vi "Lambda Genesys Initialization VI.vi"(8 "error in (no error)":errorcluster, 10 "Custom XML":string, 11 "Device Item Ref in":T1 format="%.0x") -> (0 "error out":errorcluster, 3 "Device Item Ref out":T1 format="%.0x")   [LabVIEW 2011, in "Lambda Genesys2 Custom Device.lvlib"]
doc: "The Initialization VI is used to populate the tree with the most important elements. It is mandatory to add at least the main page!\nBy calling the Add Items VI make sure that sections are added before the channels. Also make sure that for nested sections each individual section is created (from top to bottwom)."
uses:
  Lambda Genesys2 Custom Device.lvlib
  <vilib>/NI Veristand/Custom Device API/Custom Device Item Ref.ctl
  <vilib>/NI Veristand/Custom Device API/Custom Device Channel.ctl
  <vilib>/NI Veristand/Custom Device API/Custom Device Channel Type.ctl
  <vilib>/NI Veristand/Custom Device API/Custom Device Loop Type.ctl
  Lambda Genesys Device Properties.vi
  <vilib>/NI Veristand/Custom Device API/Set Item Property (String).vi
  <vilib>/NI Veristand/Custom Device API/Set Item Property (I32).vi
  <vilib>/NI Veristand/Custom Device API/Custom Device API.lvlib
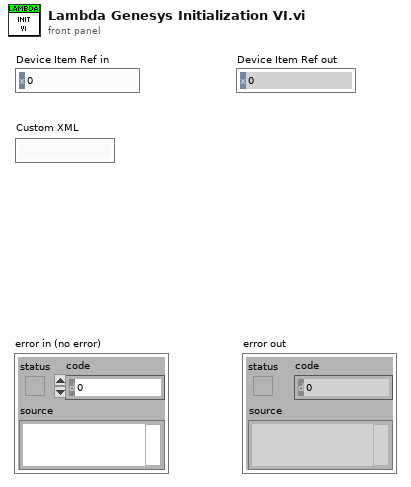
[diagram p1: front panel]
types:
  T1 = typedef "Custom Device API.lvlib/Custom Device Item Ref.ctl" = u64
  T2 = typedef "Custom Device API.lvlib/Custom Device Channel.ctl" = cluster{"Type":T3, "Units":string, "Default Value":dbl, "Faultable":bool, "Scalable":bool}
  T3 = typedef "Custom Device API.lvlib/Custom Device Channel Type.ctl" = enum16{"Input", "Output"}
  T4 = typedef "Custom Device API.lvlib/Custom Device Loop Type.ctl" = enum32{"While Loop", "Timed Loop"}
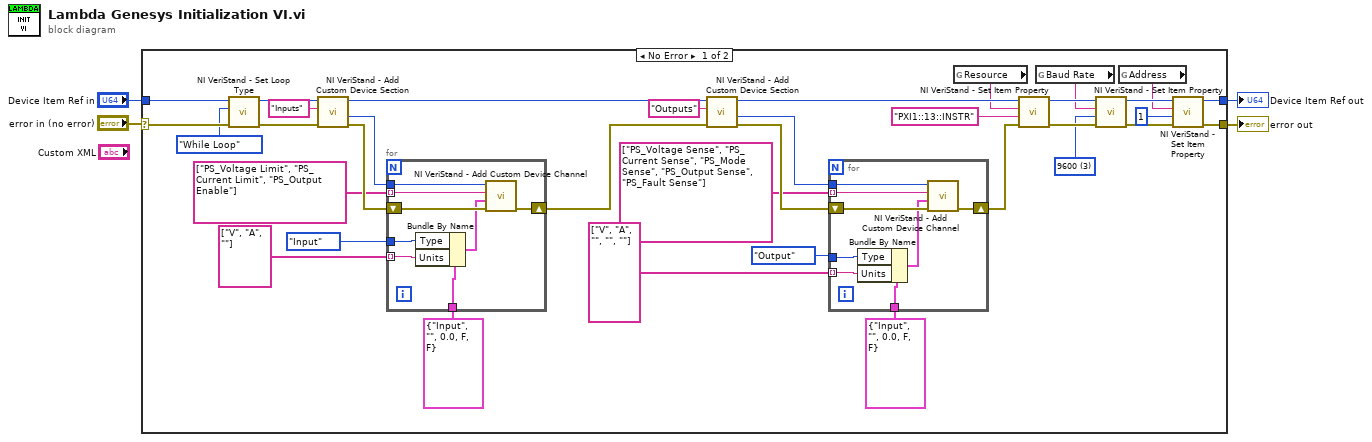
[diagram p0: block diagram]
diagram:
  n1 = case shown="No Error" "error in (no error)" {
    selector: "error in (no error)" -> [w37 w57]
    tunnel: [w7 w57] -> w2
    tunnel: "Device Item Ref in" -> [w17 w56]
    tunnel: [w6 w56] -> w1
    frame No Error {
      w10 = 3 items=["1200", "2400", "4800", "9600", "19200"] ("Baud Rate")
      n2 = call <vilib>:"NI VeriStand - Set Loop Type.vi"("error in (no error)"=w37, "Loop type"=Custom_Device_Loop_Type."While Loop", "Device Ref in"=w17) -> ("error out"=w35:errorcluster, "Device Ref out"=w33:T1)  [unwired: 1 in, 6 out]
      n3 = call <vilib>:"NI VeriStand - Add Custom Device Section.vi"("error in (no error)"=w35, "Section Name"="Inputs", "Parent Ref in"=w33) -> ("error out"=w31:errorcluster, "Section Ptr"=w32:T1, "Parent Ref out"=w25:T1)  [unwired: 4 in, 2 out]
      n4 = for {
        tunnel: w32 -> [w54]
        shift-right: [w48] -> w24
        shift-left: w31 -> [w55]
        tunnel: string[] ["PS_Voltage Limit", "PS_Current Limit", "PS_Output Enable"] -> [w53] mode=indexing
        tunnel: T2 {"Type"=enum."Input", "Units"="", "Default Value"=0.0, "Faultable"=FALSE, "Scalable"=FALSE} ("Channel") -> [w52]
        tunnel: Custom_Device_Channel_Type."Input" ("Type") -> [w51]
        tunnel: string[] ["V", "A", ""] -> [w50] mode=indexing
        n5 = Bundle By Name(cluster=w52, "Type"=w51, "Units"=w50) -> (w49:T2)
        n6 = call <vilib>:"NI VeriStand - Add Custom Device Channel.vi"("error in (no error)"=w55, "Channel"=w49, "Channel Name"=w53, "Parent Ref in"=w54) -> ("error out"=w48:errorcluster)  [unwired: 4 in, 3 out]
      }
      n7 = call <vilib>:"NI VeriStand - Add Custom Device Section.vi"("error in (no error)"=w24, "Section Name"="Outputs", "Parent Ref in"=w25) -> ("error out"=w23:errorcluster, "Section Ptr"=w22:T1, "Parent Ref out"=w16:T1)  [unwired: 4 in, 2 out]
      n8 = for {
        tunnel: w22 -> [w46]
        shift-right: [w40] -> w15
        shift-left: w23 -> [w47]
        tunnel: string[] ["PS_Voltage Sense", "PS_Current Sense", "PS_Mode Sense", "PS_Output Sense", "PS_Fault Sense"] -> [w45] mode=indexing
        tunnel: T2 {"Type"=enum."Input", "Units"="", "Default Value"=0.0, "Faultable"=FALSE, "Scalable"=FALSE} ("Channel") -> [w44]
        tunnel: Custom_Device_Channel_Type."Output" ("Type") -> [w43]
        tunnel: string[] ["V", "A", "", "", ""] -> [w42] mode=indexing
        n9 = Bundle By Name(cluster=w44, "Type"=w43, "Units"=w42) -> (w41:T2)
        n10 = call <vilib>:"NI VeriStand - Add Custom Device Channel.vi"("error in (no error)"=w47, "Channel"=w41, "Channel Name"=w45, "Parent Ref in"=w46) -> ("error out"=w40:errorcluster)  [unwired: 4 in, 3 out]
      }
      n11 = global read "Lambda Genesys Device Properties.vi" "Resource"() -> (w14:string)
      n12 = call-poly <vilib>:"NI VeriStand - Set Item Property.vi"("error in (no error)"=w15, "Value"="PXI1::13::INSTR", "Property Name"=w14, "Item Ref in"=w16) -> ("error out"=w11:errorcluster, "Item Ref out"=w38:T1)  [unwired: 6 out]
      n13 = global read "Lambda Genesys Device Properties.vi" "Baud Rate"() -> (w12:string)
      n14 = call-poly <vilib>:"NI VeriStand - Set Item Property.vi"("error in (no error)"=w11, "Value"=w10, "Property Name"=w12, "Item Ref in"=w38) -> ("error out"=w8:errorcluster, "Item Ref out"=w39:T1)  [unwired: 6 out]
      n15 = global read "Lambda Genesys Device Properties.vi" "Address"() -> (w9:string)
      n16 = call-poly <vilib>:"NI VeriStand - Set Item Property.vi"("error in (no error)"=w8, "Value"=1, "Property Name"=w9, "Item Ref in"=w39) -> ("error out"=w7:errorcluster, "Item Ref out"=w6:T1)  [unwired: 6 out]
    }
    frame Error {
    }
  }
  "Device Item Ref out" <- w1
  "error out" <- w2
